vi "Vision Processing.vi"(4 "error in (no error)":errorcluster, 7 "Image Size":T3=enum."320x240") -> ()   [LabVIEW 2013]
doc: "This VI runs in parallel to other tasks. It gets images from the camera, processes them for color or shape and use that information to affect robot behavior."
uses:
  <vilib>/Rock Robotics/WPI/Camera/WPI_CameraImageSize.ctl
  Example_Code/2014 Target Detection/TargetType.ctl
  <vilib>/Rock Robotics/WPI/Camera/WPI_CameraWhite Balance Values.ctl
  <vilib>/Rock Robotics/WPI/Camera/WPI_CameraExposure Values.ctl
  <vilib>/Rock Robotics/WPI/Camera/WPI_CameraFrameRate.ctl
  Robot Global Data.vi
panel:
  in  "Score cutoff":dbl=50.0
  out "Loop time (ms)":u32
  out "Distance (ft)":dbl
  out "Scores.State":T1
  in  "Color Components":T2={"Hue"={100.0, 201.0}, "Sat"={0.0, 255.0}, "Val"={234.0, 255.0}} {"Val" scale=0.0..255.0; "Sat" scale=0.0..255.0; "Hue" scale=0.0..255.0 scale format="%#_3g"}
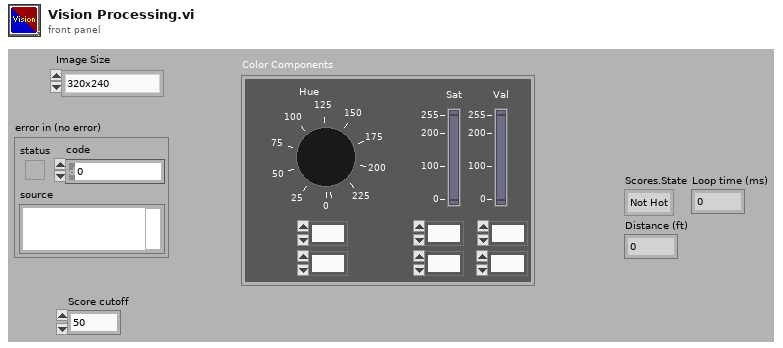
[diagram p1: front panel]
types:
  T1 = typedef "TargetType.ctl" = enum16{"Not Hot", "Hot"}
  T2 = cluster{"Hue":cluster{dbl, dbl}, "Sat":cluster{dbl, dbl}, "Val":cluster{dbl, dbl}}
  T3 = typedef "WPI_CameraImageSize.ctl" = enum16{"640x480", "320x240", "160x120"}
  T4 = typedef "WPI_CameraFrameRate.ctl" = u32
  T5 = typedef "WPI_CameraExposure Values.ctl" = enum16{"Auto", "Flicker-free 50 Hz", "Flicker-free 60 Hz", "Hold current"}
  T6 = typedef "WPI_CameraWhite Balance Values.ctl" = enum16{"Auto", "Fixed indoor", "Fixed outdoor 1", "Fixed outdoor 2", "Fixed fluorescent 1", "Fixed fluorescent 2", "Hold current"}
  T7 = typedef "Image Type" = u32
  T8 = typedef "WPI_CameraDevRef.ctl" = cluster{"Camera Address":string, "CameraStatus":errorcluster, "Acquire Image Notifier":refnum<notifier>}
  T9 = typedef "IMAQ Image.ctl" = refnum<image>
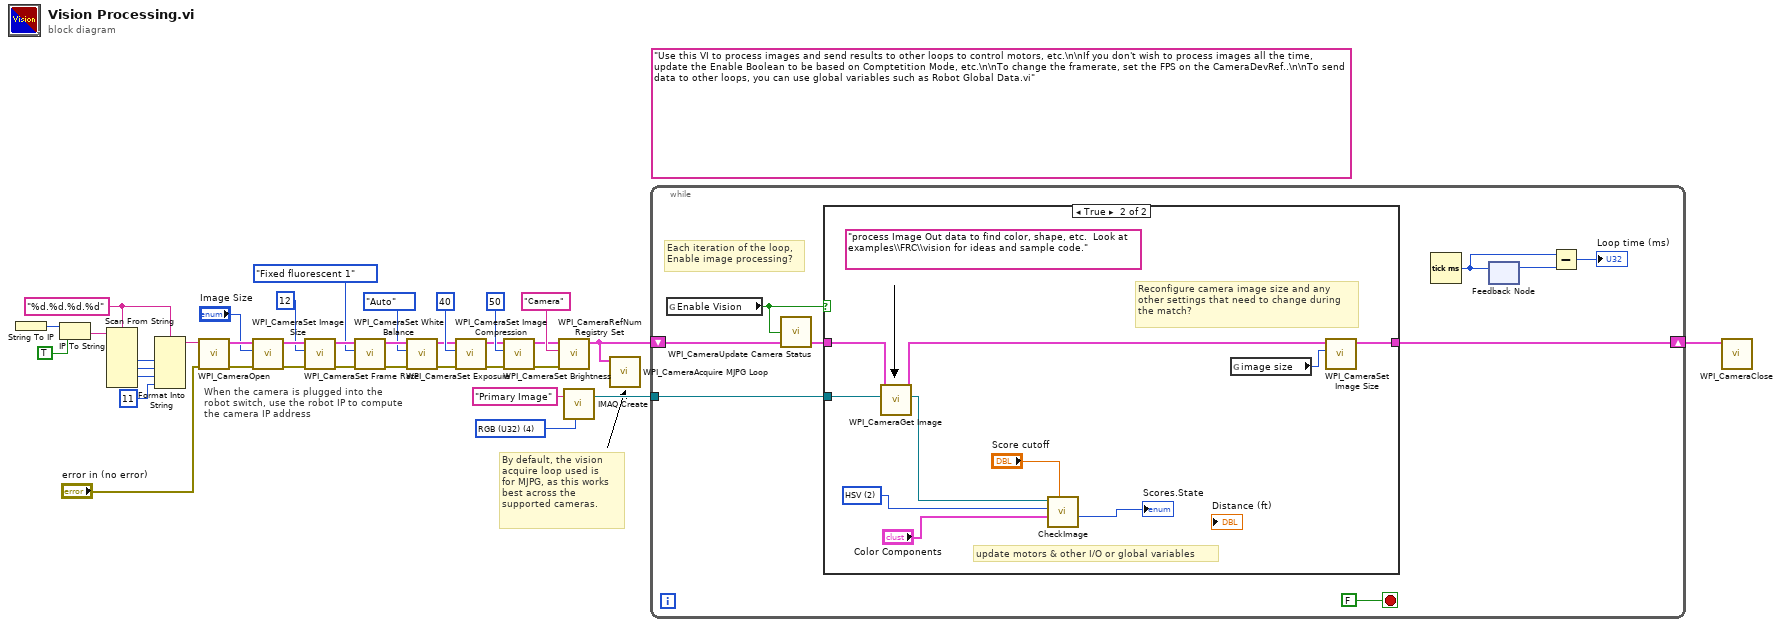
[diagram p0: block diagram]
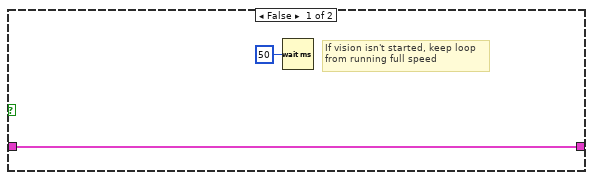
[diagram p2: hidden frame]
diagram:
  w6 = "%d.%d.%d.%d" ("format string")
  (unwired) "Use this VI to process images and send results to other loops to control motors, etc.\n\nIf you don't wish to process images all the time, update the Enable Boolean to be based on Comptetition Mode, etc.\n\nTo change the framerate, set the FPS on the CameraDevRef..\n\nTo send data to other loops, you can use global variables such as Robot Global Data.vi"
  w36 = T7 4 items=["Grayscale (U8)", "Grayscale (I16)", "Grayscale (SGL)", "Complex (CSG)", "RGB (U32)", "HSL (U32)", "RGB (U64)"] ("Image Type")
  # "When the camera is plugged into the\nrobot switch, use the robot IP to compute\nthe camera IP address"
  # "By default, the vision\nacquire loop used is\nfor MJPG, as this works\nbest across the\nsupported cameras."
  n1 = String To IP() -> (0:w13:u32)  [unwired: 1 in]
  n2 = IP To String(1:TRUE ("dot notation? (F)"), 2:w13) -> (0:w11:string)
  n3 = Scan From String(format string=w6, input string=w11) -> (output 1=w10:i32, output 2=w9:i32, output 3=w8:i32)  [unwired: 7 in, 3 out]
  n4 = Format Into String(format string=w6, w10, w9, w8, 11 ("Compression")) -> (resulting string=w5:string)  [unwired: 2 in, 1 out]
  n5 = call <vilib>:"WPI_CameraOpen.vi"("error in (no error)"="error in (no error)", "Camera Address"=w5) -> ("error out"=w24:errorcluster, "CameraDevRef"=w25:T8)  [unwired: 8 out]
  n6 = call <vilib>:"WPI_CameraSet Image Size.vi"("error in (no error)"=w24, "Image Size"="Image Size", "CameraDevRef"=w25) -> ("error out"=w23:errorcluster, "CameraDevRef Out"=w26:T8)  [unwired: 7 out]
  n7 = call <vilib>:"WPI_CameraSet Frame Rate.vi"("error in (no error)"=w23, "Frame Rate (fps)"=T4 12, "CameraDevRef"=w26) -> ("error out"=w22:errorcluster, "CameraDevRef Out"=w28:T8)  [unwired: 7 out]
  n8 = call <vilib>:"WPI_CameraSet White Balance.vi"("error in (no error)"=w22, "White Balance"=WPI_CameraWhite_Balance_Values."Fixed fluorescent 1", "CameraDevRef"=w28) -> ("error out"=w21:errorcluster, "CameraDevRef Out"=w27:T8)  [unwired: 7 out]
  n9 = call <vilib>:"WPI_CameraSet Exposure.vi"("error in (no error)"=w21, "Exposure"=WPI_CameraExposure_Values."Auto", "CameraDevRef"=w27) -> ("error out"=w20:errorcluster, "CameraDevRef Out"=w30:T8)  [unwired: 7 out]
  n10 = call <vilib>:"WPI_CameraSet Image Compression.vi"("error in (no error)"=w20, "Compression"=40, "CameraDevRef"=w30) -> ("error out"=w19:errorcluster, "CameraDevRef Out"=w29:T8)  [unwired: 7 out]
  n11 = call <vilib>:"WPI_CameraSet Brightness.vi"("error in (no error)"=w19, "Brightness"=50, "CameraDevRef"=w29) -> ("error out"=w17:errorcluster, "CameraDevRef Out"=w18:T8)  [unwired: 7 out]
  n12 = call <vilib>:"WPI_CameraRefNum Registry Set.vi"("error in (no error)"=w17, "refnum name"="Camera", "CameraDevRef"=w18) -> ("CameraDevRef"=w4:T8)  [unwired: 8 out]
  n13 = call "IMAQ Create"("Image Name"="Primary Image", "Image Type"=w36) -> ("New Image"=w34:T9)  [unwired: 2 in, 2 out]
  n14 = call <vilib>:"WPI_CameraAcquire MJPG Loop.vi"("CameraDevRef"=w4) -> ()  [unwired: 11 in]
  n15 = while {
    shift-right: [w44] -> w2
    shift-left: w4 -> [w42]
    tunnel: w34 -> [w43]
    stop <- FALSE stop-if-true
    # "Each iteration of the loop,\nEnable image processing?"
    n16 = global read "Robot Global Data.vi" "Enable Vision"() -> (w40:bool)
    n17 = call <vilib>:"WPI_CameraUpdate Camera Status.vi"("CameraDevRef In"=w42, "Enable Vision"=w40) -> ("CameraDevRef Out"=w41:T8)  [unwired: 3 in]
    n18 = case shown="True" w40 {
      tunnel: w43 -> [_ w56]
      tunnel: [w47 w57] -> w44
      tunnel: w41 -> [w47 w54]
      frame False {
        # "If vision isn't started, keep loop\nfrom running full speed"
        n19 = Wait (ms)(milliseconds to wait=u32 50) -> ()  [unwired: 1 out]
      }
      frame True {
        w49 = u16 2 items=["RGB", "HSL", "HSV", "HSI"] ("Color System")
        (unwired) "process Image Out data to find color, shape, etc.  Look at examples\\FRC\\vision for ideas and sample code."
        # "update motors & other I/O or global variables"
        # "Reconfigure camera image size and any\nother settings that need to change during\nthe match?"
        n20 = call <vilib>:"WPI_CameraGet Image.vi"("Image"=w56, "CameraDevRef"=w54) -> ("Image Out"=w51:T9, "CameraDevRef Out"=w53:T8)  [unwired: 1 in, 7 out]
        n21 = call "CheckImage.vi"("Score cutoff"="Score cutoff", "Color Components"="Color Components", "Color System"=w49, "Image"=w51) -> ("Scores.State"=→"Scores.State":T1)  [unwired: 4 in, 3 out]
        n22 = global read "Robot Global Data.vi" "image size"() -> (w55:T3)
        n23 = call <vilib>:"WPI_CameraSet Image Size.vi"("Image Size"=w55, "CameraDevRef"=w53) -> ("CameraDevRef Out"=w57:T8)  [unwired: 1 in, 8 out]
      }
    }
    n24 = Tick Count (ms)() -> (millisecond timer value=w38:u32)
    n25 = feedback-in #1(w38) -> ()
    n26 = feedback #1() -> (w39:u32)  [unwired: 1 in]
    n27 = Subtract(x=w38, y=w39) -> (x-y=→"Loop time (ms)":u32)
  }
  n28 = call <vilib>:"WPI_CameraClose.vi"("CameraDevRef"=w2) -> ()  [unwired: 1 in, 10 out]
